vi "get_all_experimental_folders_given_date.vi"(8 "error in":errorcluster, 11 "Date (YYYYMMDD)":string) -> (0 "error out":errorcluster, 3 "Expeirment Folders":string[](array[string]))   [LabVIEW 2019]
uses:
  ParametersGlobal.vi
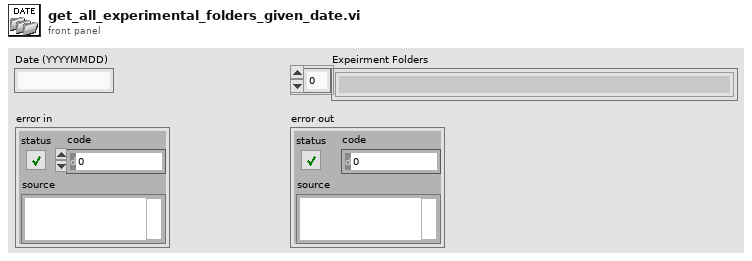
[diagram p1: front panel]
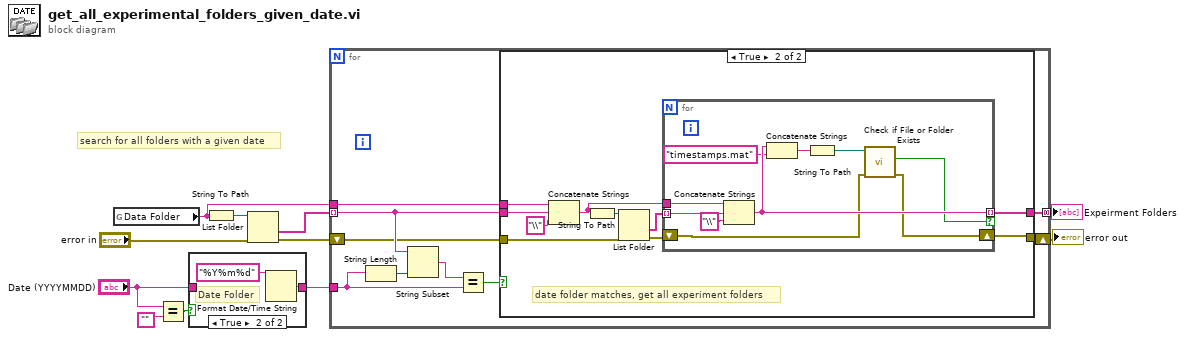
[diagram p0: block diagram]
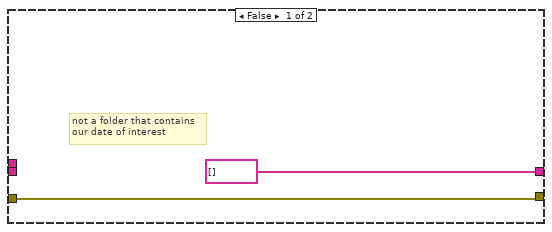
[diagram p3: hidden frame]
diagram:
  # "search for all folders with a given date"
  n1 = global read "ParametersGlobal.vi" "Data Folder"() -> (w5:string)
  n2 = Equal?(x="Date (YYYYMMDD)", y="") -> (x = y?=w6:bool)
  n3 = case shown="True" w6 {
    tunnel: [w12 w13] -> w8
    tunnel: "Date (YYYYMMDD)" -> [w12 _]
    frame False {
    }
    frame True {
      # "Date Folder"
      n4 = Format Date/Time String(time format string (%c)="%Y%m%d") -> (date/time string=w13:string)  [unwired: 2 in]
    }
  }
  n5 = String To Path(string=w5) -> (path=w11:path)
  n6 = List Folder(path=w11, error in="error in") -> (folder names=w10:string[], error out=w4:errorcluster)  [unwired: 2 in, 2 out]
  n7 = for {
    tunnel: w10 -> [w19] mode=indexing
    tunnel: w8 -> [w21]
    tunnel: w5 -> [w18]
    shift-right: [w16] -> w2
    shift-left: w4 -> [w17]
    tunnel: [w15] -> w3 mode=concatenating
    n8 = String Length(string=w21) -> (length=w23:i32)
    n9 = String Subset(string=w19, length (rest)=w23) -> (substring=w22:string)  [unwired: 1 in]
    n10 = Equal?(x=w22, y=w21) -> (x = y?=w20:bool)
    n11 = case shown="True" w20 {
      tunnel: w19 -> [_ w34]
      tunnel: w18 -> [_ w35]
      tunnel: w17 -> [w24 w31]
      tunnel: [w24 w26] -> w16
      tunnel: [string[] [] w28] -> w15
      frame False {
        # "not a folder that contains\nour date of interest"
      }
      frame True {
        # "date folder matches, get all experiment folders"
        n12 = Concatenate Strings(w35, w34, "\\" ("string")) -> (w29:string)
        n13 = String To Path(string=w29) -> (path=w32:path)
        n14 = List Folder(path=w32, error in=w31) -> (folder names=w30:string[], error out=w27:errorcluster)  [unwired: 2 in, 2 out]
        n15 = for {
          tunnel: w30 -> [w44] mode=indexing
          tunnel: w29 -> [w45]
          tunnel: [w42] -> w28 mode=indexing if=w36
          shift-right: [w37] -> w26
          shift-left: w27 -> [w38]
          n16 = Concatenate Strings(w45, w44, "\\" ("string")) -> (w42:string)
          n17 = Concatenate Strings(w42, "timestamps.mat" ("string")) -> (w40:string)
          n18 = String To Path(string=w40) -> (path=w39:path)
          n19 = call <vilib>:"Check if File or Folder Exists.vi"("error in (no error)"=w38, "path"=w39) -> ("error out"=w37:errorcluster, "file or folder exists?"=w36:bool)  [unwired: 7 in, 1 out]
        }
      }
    }
  }
  "Expeirment Folders" <- w3
  "error out" <- w2
